vi "Create Directory for Dependent Items.vi"(0 "Old Main Path":path, 5 "Old Dependency Path":path, 7 "New Dir":path, 11 "error in (no error)":errorcluster) -> (4 "Directory":path, 15 "error out":errorcluster)   [LabVIEW 2021, in "Path Functions.lvlib"]
uses:
  Path Functions.lvlib
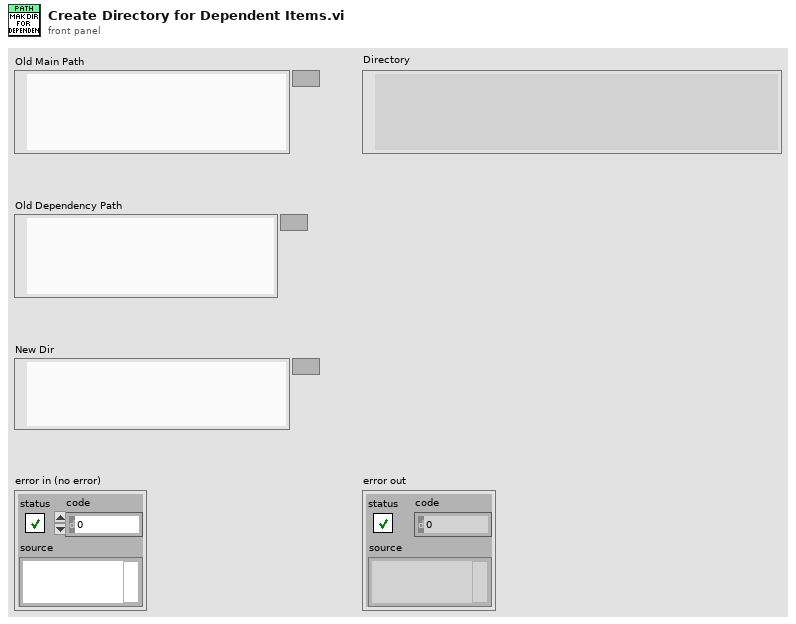
[diagram p1: front panel]
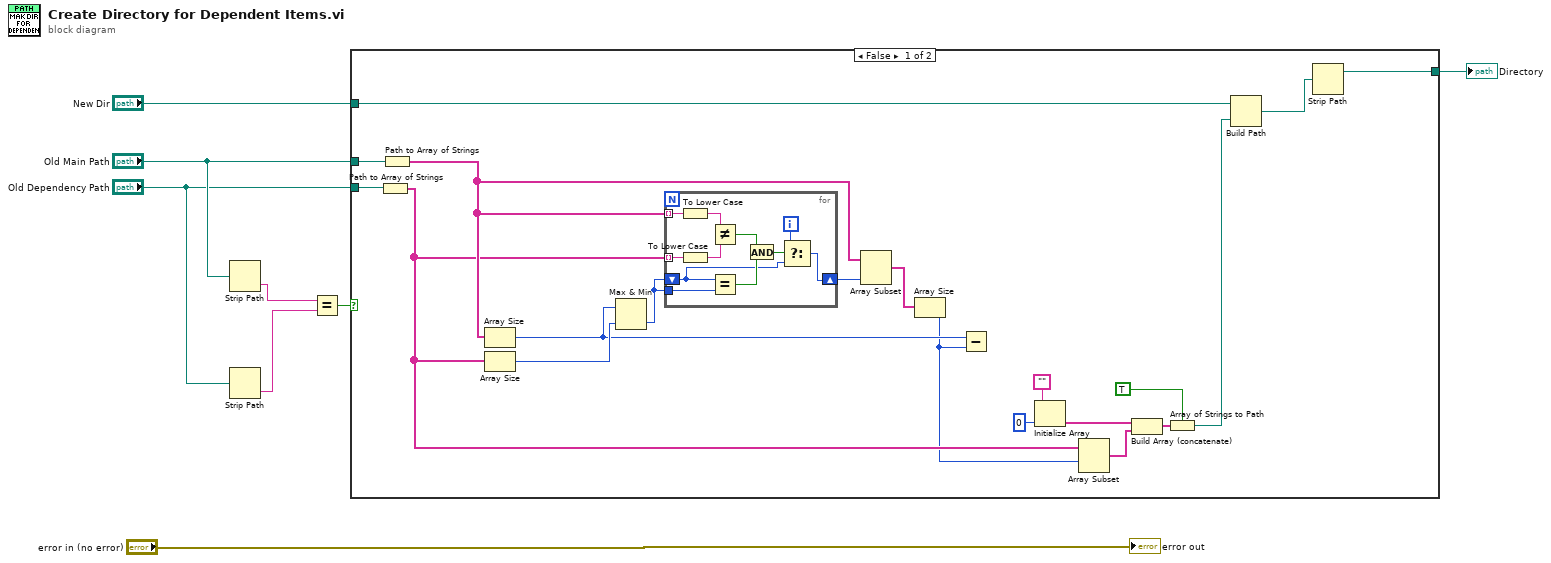
[diagram p0: block diagram]
diagram:
  n1 = Strip Path(path="Old Main Path") -> (name=w3:string)  [unwired: 1 out]
  n2 = Strip Path(path="Old Dependency Path") -> (name=w2:string)  [unwired: 1 out]
  n3 = Equal?(x=w3, y=w2) -> (x = y?=w1:bool)
  n4 = case shown="False" w1 {
    tunnel: "New Dir" -> [w28 w40]
    tunnel: [w26 w40] -> w7
    tunnel: "Old Main Path" -> [w10 _]
    tunnel: "Old Dependency Path" -> [w9 _]
    frame False {
      n5 = Path to Array of Strings(0:w9) -> (2:w18:string[])  [unwired: 1 out]
      n6 = Path to Array of Strings(0:w10) -> (2:w21:string[])  [unwired: 1 out]
      n7 = Array Size(array=w21) -> (size(s)=w23:i32)
      n8 = Array Size(array=w18) -> (size(s)=w24:i32)
      n9 = Max & Min(x=w23, y=w24) -> (min(x,y)=w25:i32)  [unwired: 1 out]
      n10 = for {
        tunnel: w21 -> [w39] mode=indexing
        tunnel: w18 -> [w38] mode=indexing
        shift-right: [w31] -> w22
        shift-left: w25 -> [w32]
        tunnel: w25 -> [w37]
        i -> [w33]
        n11 = To Lower Case(string=w39) -> (all lower case string=w30:string)
        n12 = To Lower Case(string=w38) -> (all lower case string=w29:string)
        n13 = Not Equal?(x=w30, y=w29) -> (x != y?=w35:bool)
        n14 = Equal?(x=w32, y=w37) -> (x = y?=w36:bool)
        n15 = And(x=w35, y=w36) -> (x .and. y?=w34:bool)
        n16 = Select(t=w33, s=w34, f=w32) -> (s? t:f=w31:i32)
      }
      n17 = Array Subset(array=w21, length=w22) -> (w13:string[])  [unwired: 1 in]
      n18 = Array Size(array=w13) -> (size(s)=w12:i32)
      n19 = Subtract(x=w23, y=w12) -> ()  [unwired: 1 out]
      n20 = Initialize Array("", 0 ("dimension size")) -> (w16:string[])
      n21 = Array Subset(array=w18, index=w12) -> (w19:string[])  [unwired: 1 in]
      n22 = Build Array (concatenate)(w16, w19) -> (w20:string[])
      n23 = Array of Strings to Path(0:w20, 1:TRUE ("relative")) -> (2:w14:path)
      n24 = Build Path(base path=w28, name or relative path=w14) -> (appended path=w27:path)
      n25 = Strip Path(path=w27) -> (stripped path=w26:path)  [unwired: 1 out]
    }
    frame True {
    }
  }
  "Directory" <- w7
  "error out" <- "error in (no error)"
